vi "PlotSpectrum.vi"() -> ()   [LabVIEW 2018]
panel:
  in  "Add Signal Path":string
  out "BandWidth  Power":dbl
  out "error out":errorcluster
  in  "error in (no error)":errorcluster
  in  "BandWidth":dbl=20.0 format="%#_13g"
  in  "Center Frequency":dbl=20.0 format="%#_13g"
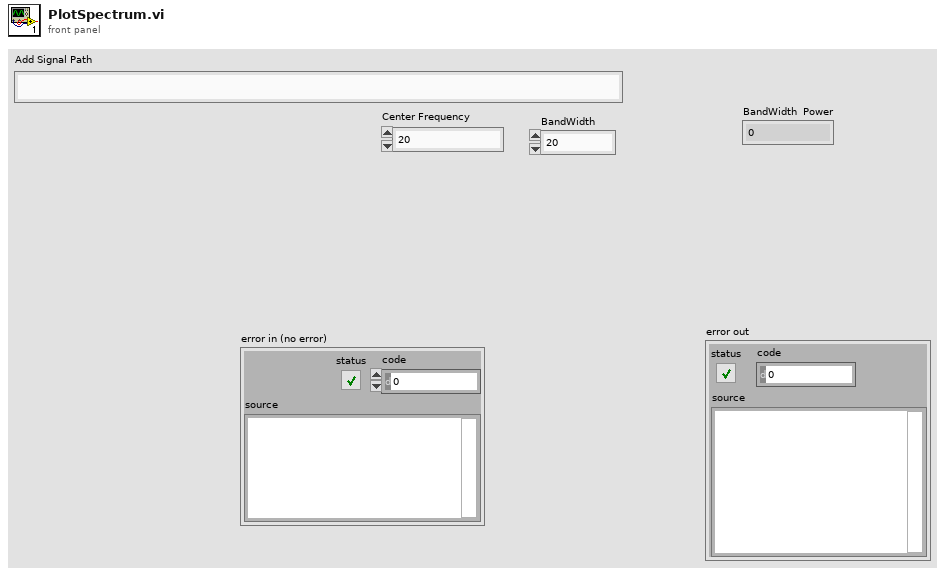
[diagram p1: front panel]
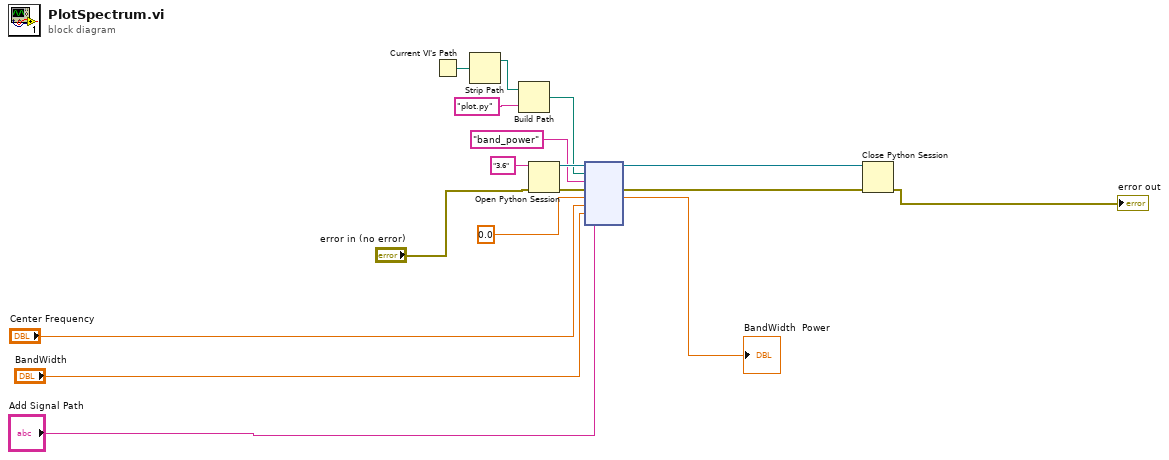
[diagram p0: block diagram]
diagram:
  n1 = Current VI's Path() -> (path=w11:path)
  n2 = Strip Path(path=w11) -> (stripped path=w10:path)  [unwired: 1 out]
  n3 = Build Path(base path=w10, name or relative path="plot.py") -> (appended path=w8:path)
  n4 = Open Python Session(python version="3.6" ("Python version"), 3:"error in (no error)") -> (session out=w17:refnum<k35>, error out=w15:errorcluster)  [unwired: 1 in]
  n5 = node(w17, w8, "band_power" ("function name"), w15, 0.0, "Center Frequency", "BandWidth", "Add Signal Path") -> (w16:refnum<k35>, w14:errorcluster, →"BandWidth  Power":dbl)  [unwired: 3 in, 2 out]
  n6 = Close Python Session(session in=w16, error in=w14) -> (11:→"error out":errorcluster)
